vi "Set Units.vi"(8 "error in":errorcluster, 10 "Units":string="mb", 11 "PPT in":refnum<class "PPT.lvclass">) -> (0 "error out":errorcluster, 3 "PPT out":refnum<class "PPT.lvclass">)   [LabVIEW 2014, in "PPT.lvclass"]
uses:
  PPT.lvclass
  PPT.lvclass/PPT.ctl
  Reusable/Session APIs/Serial/Public/Get Data/Get String.vi
  Reusable/Session APIs/Text Communication/Text Device Session.lvclass
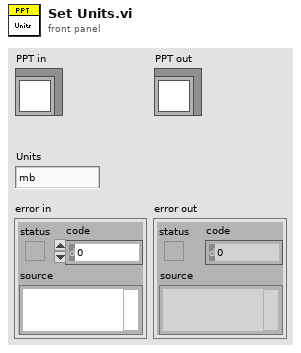
[diagram p1: front panel]
types:
  T1 = typedef "Session - Root.lvclass/Session Handle.ctl" = refnum<data-value>
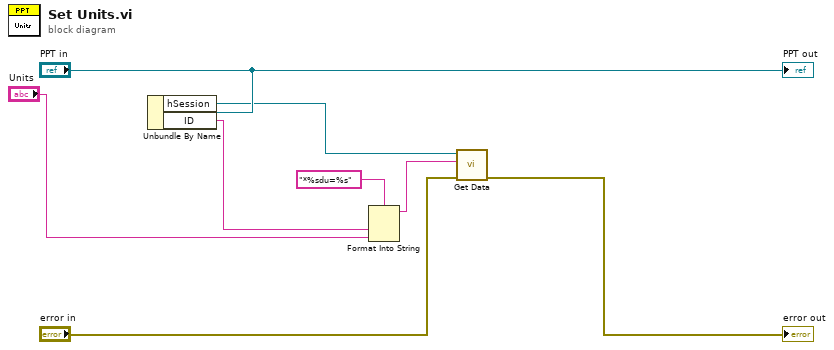
[diagram p0: block diagram]
diagram:
  n1 = Unbundle By Name("PPT in") -> ("hSession"=w7:T1, "ID"=w5:string)
  n2 = Format Into String(format string="*%sdu=%s", w5, "Units") -> (resulting string=w3:string)  [unwired: 2 in, 1 out]
  n3 = call-poly "Get Data.vi"("error in"="error in", "CMD"=w3, "handle in"=w7) -> ("error out"=→"error out":errorcluster)  [unwired: 6 in, 2 out]
  "PPT out" <- "PPT in"
